vi "pH_meter_(FPGA).vi"() -> ()   [LabVIEW 2016]
doc: "This VI will continually read single point values from 4 channels of an analog input module at a specified rate."
uses:
  <vilib>/rvi/Emulation/niFpgaGetClockAttributes.vi
  <vilib>/rvi/Emulation/niFpgaSctlEmulationGetInTimedLoop.vi
  <vilib>/rvi/Emulation/niFpgaEmulationReportErrorSimple.vi
  Instance           1 31Saved   NI 9205 Basic IO (FPGA) .vi
  <vilib>/rvi/eio/common/nirviEmuTemplateMethod_errors.vi
  <vilib>/rvi/interface/RandomDataEmulation/niFpgaRandomDataHandleErrors.vi
  <vilib>/rvi/Emulation/niFpgaCriticalErrorInLSC.vi
  <vilib>/eio/EIONode/EIONode.xnode
  <vilib>/rvi/DataTransferAndStorage/Container/XNode/niFpgaContainer.xnode
  <vilib>/rvi/interface/RandomDataEmulation/nirviRandomDataFpgaReadWriteTemplate.vi
panel:
  out "Timed Out?":bool
  out "AI0":i16
  in  "stop":bool
  in  "Loop Rate (uS)":u32
  out "FPGA\nError Out":errorcluster
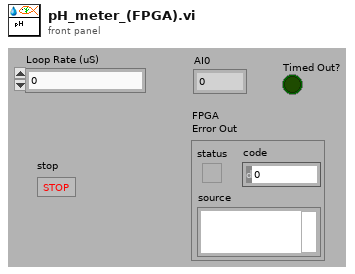
[diagram p1: front panel]
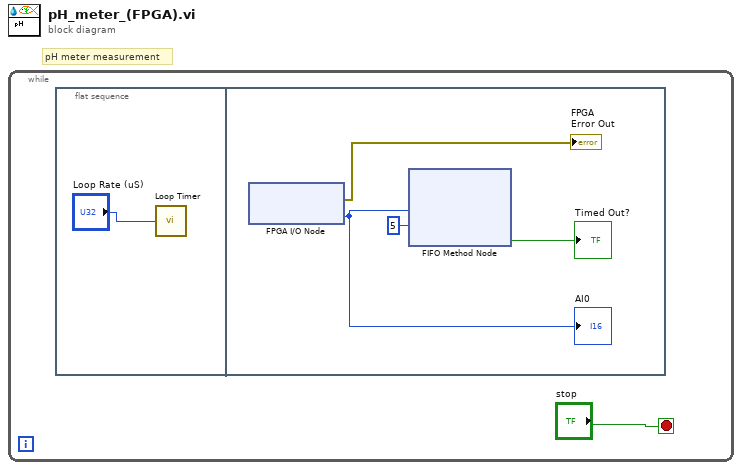
[diagram p0: block diagram]
diagram:
  # "pH meter measurement"
  n1 = while {
    stop <- "stop" stop-if-true
    n2 = flat-sequence {
      frame #0 {
        n3 = call "Loop Timer"("Count(uSec)"="Loop Rate (uS)") -> ()  [unwired: 1 out]
      }
      frame #1 {
        n4 = xnode "FPGA I/O Node"() -> ("error out"=→"FPGA\nError Out":errorcluster, "pH_Meter"=w6:i16)  [unwired: 2 in, 1 out]
        "AI0" <- w6
        n5 = xnode ("FIFO Method Node")("Element"=w6, "Timeout"=5) -> ("Timed Out?"=→"Timed Out?":bool)  [unwired: 1 in, 1 out]
      }
    }
  }
